vi "Close.vi"(8 "Error In":errorcluster, 11 "RequestMessage":refnum<class "HttpRequestMessage.lvclass">) -> (0 "Error Out":errorcluster)   [LabVIEW 2018, in "HttpClient_NET.lvlib" / "HttpRequestMessage.lvclass"]
uses:
  HttpRequestMessage.lvclass
  HttpRequestMessage.lvclass/HttpRequestMessage.ctl
  System.Net.Http
  Accessors/Read NET_HttpRequestMessage.vi
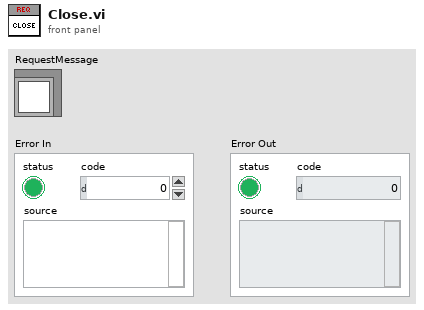
[diagram p1: front panel]
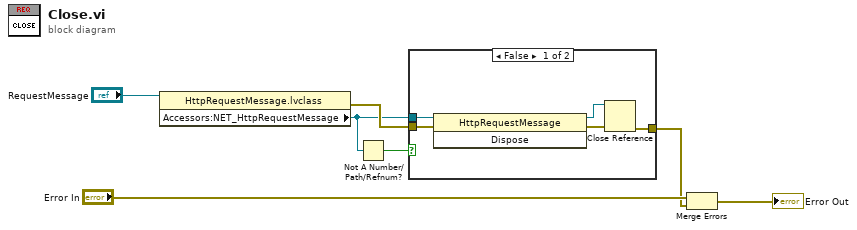
[diagram p0: block diagram]
diagram:
  n1 = property class="HttpRequestMessage.lvclass"(reference="RequestMessage") -> (error out=w3:errorcluster, "Accessors:NET_HttpRequestMessage"=w2:refnum<k24>)  [unwired: 1 in, 1 out]
  n2 = Not A Number/Path/Refnum?(number/path/refnum=w2) -> (NaN/Path/Refnum?=w1:bool)
  n3 = case shown="False" w1 {
    tunnel: [w10 w13] -> w5
    tunnel: w3 -> [w9 w13]
    tunnel: w2 -> [w8 _]
    frame False {
      n4 = invoke class="HttpRequestMessage" method="Dispose"(reference=w8, error in=w9) -> (reference out=w11:refnum<k24>, error out=w12:errorcluster)  [unwired: 1 in, 1 out]
      n5 = Close Reference(reference=w11, error in (no error)=w12) -> (error out=w10:errorcluster)
    }
    frame True {
    }
  }
  n6 = Merge Errors("Error In", w5) -> (→"Error Out":errorcluster)
